vi "Write LstBox Refnum.vi"(8 "error in (no error)":errorcluster, 10 "LstBox Refnum":refnum<vi>, 11 "Test Selector in":refnum<class "Test Selector.lvclass">) -> (0 "error out":errorcluster, 3 "Test Selector out":refnum<class "Test Selector.lvclass">)   [LabVIEW 2019, in "Test Selector.lvlib" / "Test Selector.lvclass"]
uses:
  Test Selector.lvclass
  Test Selector.lvclass/Test Selector.ctl
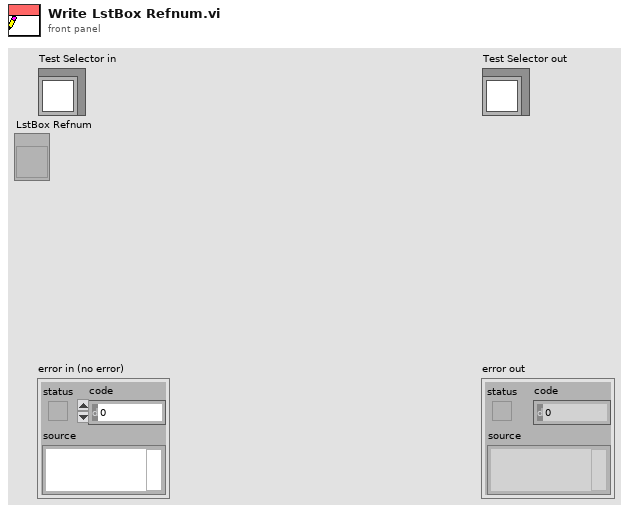
[diagram p1: front panel]
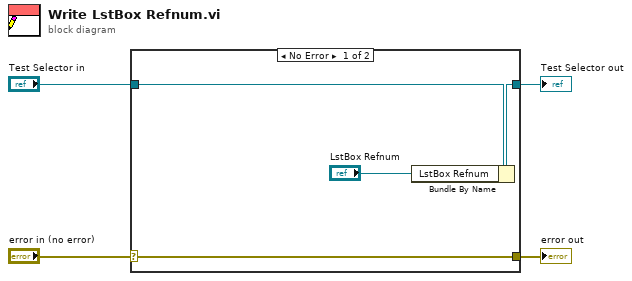
[diagram p0: block diagram]
diagram:
  n1 = case shown="No Error" "error in (no error)" {
    selector: "error in (no error)" -> [w8 w9]
    tunnel: [w8 w9] -> w3
    tunnel: [w6 w10] -> w1
    tunnel: "Test Selector in" -> [w7 w10]
    frame No Error {
      n2 = Bundle By Name(cluster=w7, "LstBox Refnum"="LstBox Refnum") -> (w6:refnum<class "Test Selector.lvclass">)
    }
    frame Error {
    }
  }
  "error out" <- w3
  "Test Selector out" <- w1
